vi "GUID_EditVI.vi"() -> ()   [LabVIEW 2018]
panel:
  in  "LicencePath":string="C:\\Users\\Marco Preziani\\Documents\\Help_Crypting_repository - V2.2\\Folder_xLicence\\LIC_Help_Viewer.lic"
  in  "HostIdentifier":string
  in  ".NET GUID":string="{9248297E-2DE6-4513-9AD6-2B44F4348F90}"
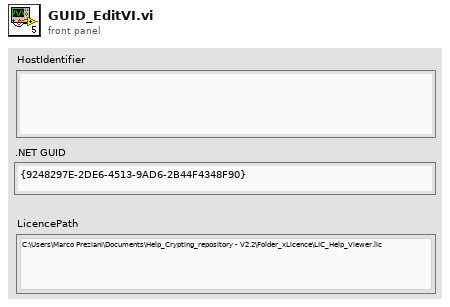
[diagram p1: front panel]
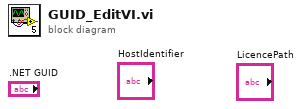
[diagram p0: block diagram]
diagram:
